vi "Read Palette info.vi"(8 "error in":errorcluster, 9 "palette type":T1=-1 items=["Functions"=-1, "Controls"=-2], 10 "palette path 2":path, 11 "palette path  1":path) -> (0 "error out":errorcluster, 1 "Palettes Different?":bool, 2 "palette data 2":T2 {"view format" items=["Icons", "Text", "Icons and Text"]}, 3 "palette data 1":T2 {"view format" items=["Icons", "Text", "Icons and Text"]})   [LabVIEW 2017]
uses:
  <vilib>/Palette API/Palette Menu/Public Type Define/Palette Data.ctl
  <vilib>/Palette API/Palette Menu/Public Type Define/View Format.ctl
  <vilib>/Palette API/Palette Menu/Public Type Define/Items.ctl
  <vilib>/Palette API/Palette Menu/Public Type Define/Item.ctl
  <vilib>/Palette API/Palette Menu/Public Type Define/Help Info.ctl
  <vilib>/Palette API/Palette Menu/Public Type Define/Synchronize Info.ctl
  <vilib>/Palette API/Palette Menu/Public Type Define/Palette type.ctl
  <vilib>/Palette API/Palette Menu/Palette Menu.lvlib
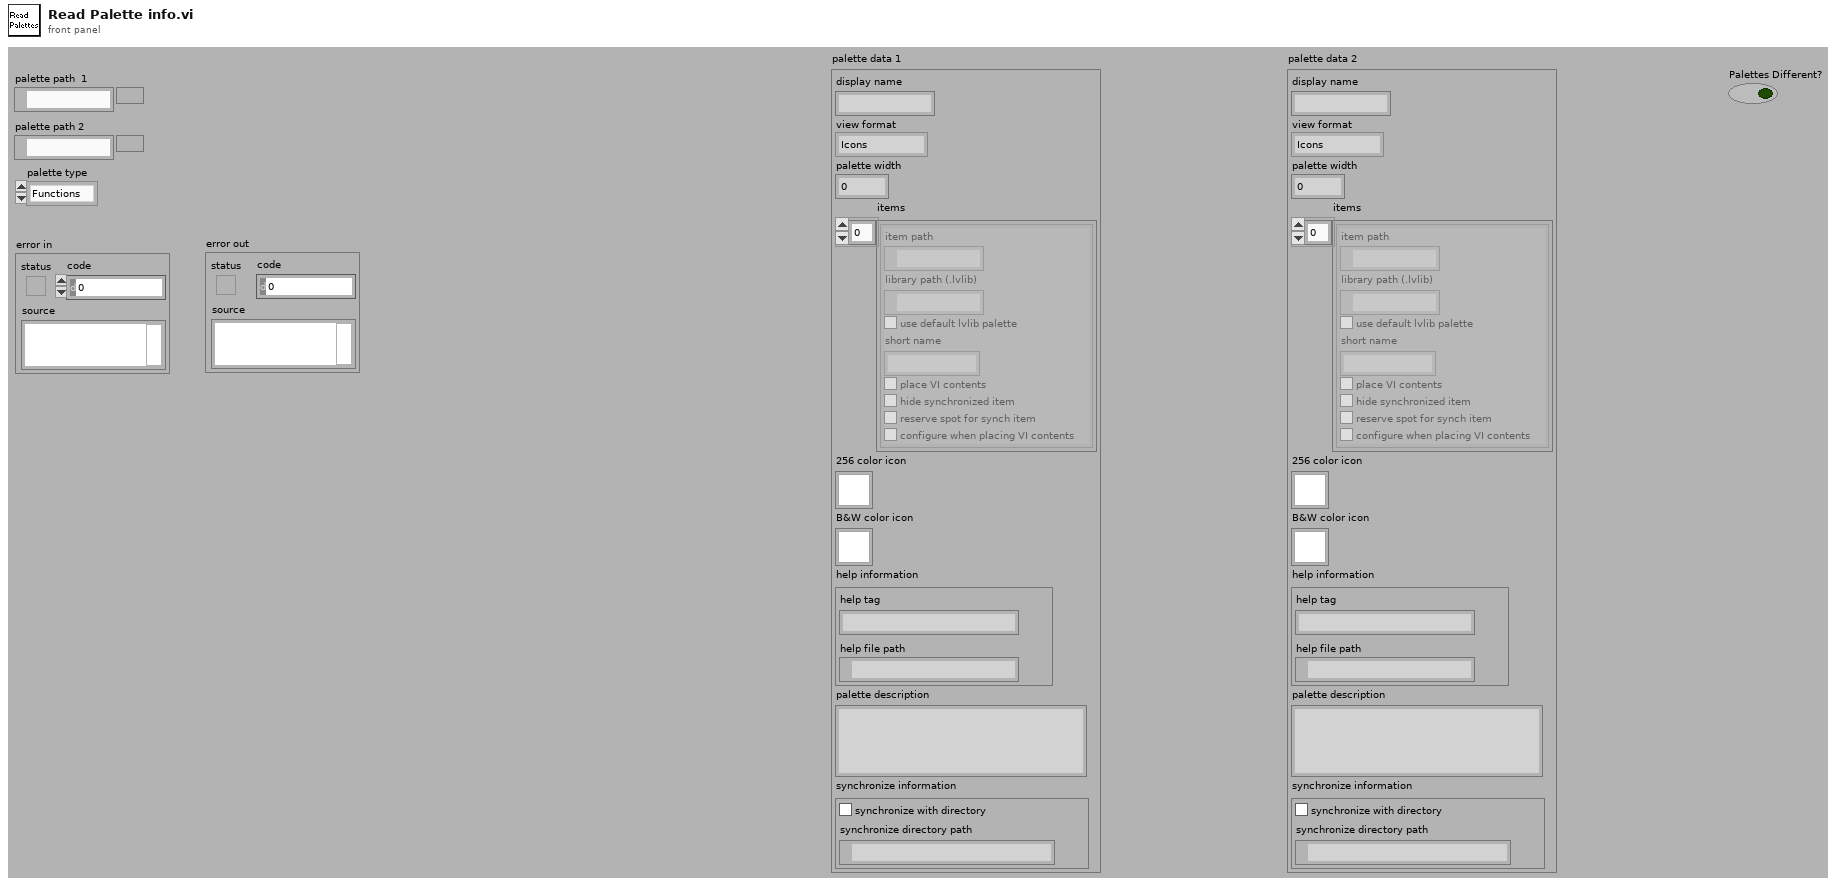
[diagram p1: front panel]
types:
  T1 = typedef "Palette Menu.lvlib/Palette type.ctl" = i32
  T2 = typedef "Palette Menu.lvlib/Palette Data.ctl" = cluster{"display name":string, "view format":T3, "palette width":i16, "items":T4, "256 color icon":picture, "B&W color icon":picture, "help information":T6, "palette description":string, "synchronize information":T7}
  T3 = typedef "Palette Menu.lvlib/View Format.ctl" = u16
  T4 = typedef "Palette Menu.lvlib/Items.ctl" = T5[]
  T5 = typedef "Palette Menu.lvlib/Item.ctl" = cluster{"item path":path, "library path (.lvlib)":path, "use default lvlib palette":bool, "short name":string, "place VI contents":bool, "hide synchronized item":bool, "reserve spot for synch item":bool, "configure when placing VI contents":bool}
  T6 = typedef "Palette Menu.lvlib/Help Info.ctl" = cluster{"help tag":string, "help file path ":path}
  T7 = typedef "Palette Menu.lvlib/Synchronize Info.ctl" = cluster{"synchronize with directory":bool, "synchronize directory path":path}
  T8 = cluster{"display name":bool, "view format":bool, "palette width":bool, "items":cluster{"item path":bool, "library path (.lvlib)":bool, "use default lvlib palette":bool, "short name":bool, "place VI contents":bool, "hide synchronized item":bool, "reserve spot for synch item":bool, "configure when placing VI contents":bool}[], "256 color icon":bool, "B&W color icon":bool, "help information":cluster{"help tag":bool, "help file path ":bool}, "palette description":bool, "synchronize information":cluster{"synchronize with directory":bool, "synchronize directory path":bool}}
  T9 = cluster{"synchronize with directory":bool, "synchronize directory path":bool}
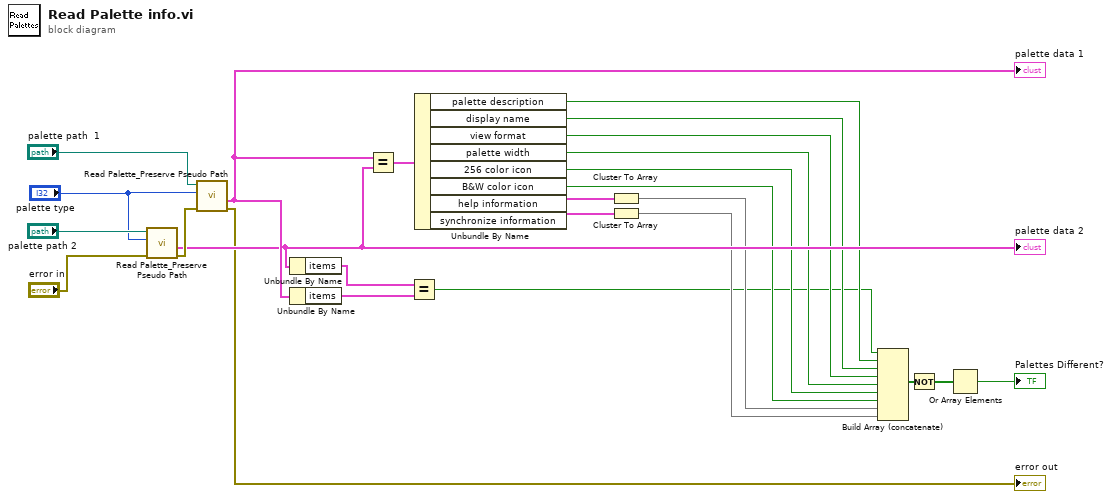
[diagram p0: block diagram]
diagram:
  n1 = call "Read Palette_Preserve Pseudo Path.vi"("error in (no error)"="error in", "palette type"="palette type", "palette path"="palette path 2") -> ("error out"=w25:errorcluster, "palette data"=w23:T2)  [unwired: 7 out]
  "palette data 2" <- w23
  n2 = call "Read Palette_Preserve Pseudo Path.vi"("error in (no error)"=w25, "palette type"="palette type", "palette path"="palette path  1") -> ("error out"=→"error out":errorcluster, "palette data"=w24:T2)  [unwired: 7 out]
  "palette data 1" <- w24
  n3 = Unbundle By Name(w23) -> ("items"=w3:T4)
  n4 = Unbundle By Name(w24) -> ("items"=w2:T4)
  n5 = Equal?(x=w24, y=w23) -> (x = y?=w13:T8)
  n6 = Equal?(x=w3, y=w2) -> (x = y?=w1:bool)
  n7 = Unbundle By Name(w13) -> ("palette description"=w9:bool, "display name"=w8:bool, "view format"=w7:bool, "palette width"=w6:bool, "256 color icon"=w5:bool, "B&W color icon"=w4:bool, "help information"=w14:cluster{"help tag":bool, "help file path ":bool}, "synchronize information"=w15:T9)
  n8 = Cluster To Array(cluster=w14) -> (array=w19:bool[])
  n9 = Cluster To Array(cluster=w15) -> (array=w20:bool[])
  n10 = Build Array (concatenate)(w1, w9, w8, w7, w6, w5, w4, w19, w20) -> (w16:bool[])
  n11 = Not(x=w16) -> (.not. x?=w18:bool[])
  n12 = Or Array Elements(Boolean array=w18) -> (logical OR=→"Palettes Different?":bool)
